vi "Condition Delete Controls.vi"(8 "error in":errorcluster, 9 "Control Terminals":i32[](array[numeric]), 10 "VI Ref":refnum<vi>) -> (0 "error out":errorcluster)   [LabVIEW 2025, in "_Rescript.lvlib" / "_Rescript.lvclass"]
uses:
  _Rescript.lvclass
  _Rescript.lvclass/_Rescript.ctl
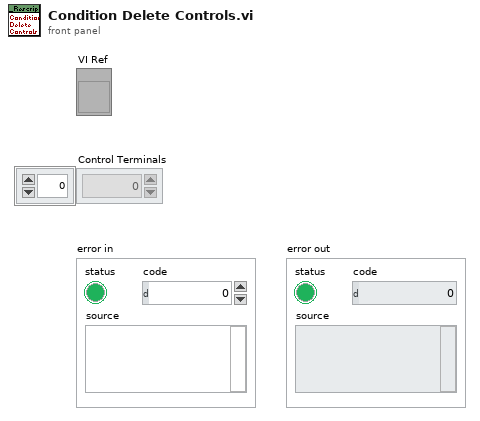
[diagram p1: front panel]
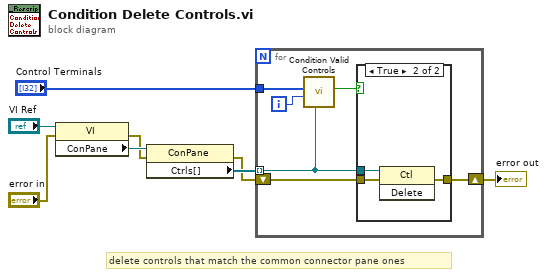
[diagram p0: block diagram]
diagram:
  # "delete controls that match the common connector pane ones"
  n1 = property class="VI"(reference="VI Ref", error in="error in") -> (error out=w5:errorcluster, "ConPane"=w8:refnum<vi>)  [unwired: 1 out]
  n2 = property class="ConPane"(reference=w8, error in=w5) -> (error out=w6:errorcluster, "Ctrls[]"=w7:refnum<vi>[])  [unwired: 1 out]
  n3 = for {
    tunnel: w7 -> [w10] mode=indexing
    shift-right: [w14] -> w2
    shift-left: w6 -> [w13]
    tunnel: "Control Terminals" -> [w12]
    i -> [w11]
    n4 = call "Condition Valid Controls.vi"("Ctl Refnum"=w10, "Terminal Index"=w11, "Control Terminals"=w12) -> ("Valid"=w9:bool)  [unwired: 8 in]
    n5 = case shown="True" w9 {
      tunnel: w10 -> [_ w18]
      tunnel: [w15 w17] -> w14
      tunnel: w13 -> [w15 w16]
      frame False {
      }
      frame True {
        n6 = invoke class="Ctl" method="Delete"(reference=w18, error in=w16) -> (error out=w17:errorcluster)  [unwired: 1 in, 2 out]
      }
    }
  }
  "error out" <- w2
